vi "MeasuringDevice.Init.vi"(8 "error in (no error)":errorcluster, 11 "OPM.ThorlabsPM400":refnum<class "OPM.ThorlabsPM400.lvclass">) -> (0 "error out":errorcluster, 3 "OPM.ThorlabsPM400 out":refnum<class "OPM.ThorlabsPM400.lvclass">)   [LabVIEW 2017, in "OPM.ThorlabsPM400.lvclass"]
doc: "---------------------------------------------------------------\nJKI State Machine Objects™\nhttp://jki.net/state-machine-objects/\nCopyright (C) 2005-2015, JKI <info@jki.net>\nALL RIGHTS RESERVEDJKI State Machine Objects (SMO) 1.0.0.5\nJKI - JKI\nCopyright (c) 2016, JKI"
uses:
  OPM.ThorlabsPM400.lvclass
  D:/upwork/Laser Measurement Tool/Laser/project/Subsystems/OPM/OPM.lvclass
  Typedefs/Resource--Cluster.ctl
  OPM/OPM.lvclass
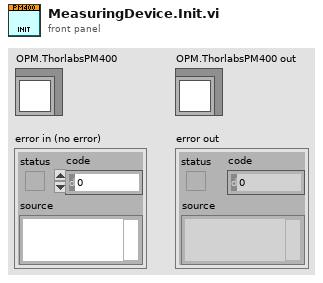
[diagram p1: front panel]
types:
  T1 = typedef "OPM.ThorlabsPM400.lvclass/Resource--Cluster.ctl" = cluster{"Instrument handle":refnum<visa-resource-name>}
  T2 = typedef "OPM.lvclass/Configuration--Cluster.ctl" = cluster{"Resource Name":string}
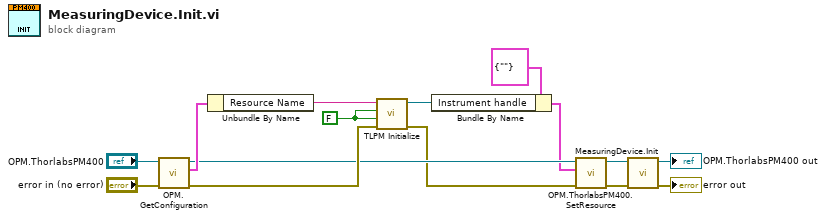
[diagram p0: block diagram]
diagram:
  w9 = FALSE ("ID Query (Do Query)")
  n1 = call "OPM.GetConfiguration.vi"("error in (no error)"="error in (no error)", "PM"="OPM.ThorlabsPM400") -> ("error out"=w8:errorcluster, "Configuration"=w11:T2, "PM out"=w5:refnum<class "OPM.ThorlabsPM400.lvclass">)  [unwired: 7 in]
  n2 = Unbundle By Name(w11) -> ("Resource Name"=w10:string)
  n3 = call <instrlib>:"TLPM Initialize.vi"("error in (no error)"=w8, "Reset Device (Reset Device)"=w9, "ID Query (Do Query)"=w9, "resource name"=w10) -> ("error out"=w3:errorcluster, "instrument handle out"=w6:refnum<visa-resource-name>)  [unwired: 6 in]
  n4 = Bundle By Name(cluster=T1 {"Instrument handle"=""} ("Resource"), "Instrument handle"=w6) -> (w4:T1)
  n5 = call "OPM.ThorlabsPM400.SetResource.vi"("error in (no error)"=w3, "Resource"=w4, "OPM.ThorlabsPM400 in"=w5) -> ("error out"=w1:errorcluster, "OPM.ThorlabsPM400 out"=w2:refnum<class "OPM.ThorlabsPM400.lvclass">)  [unwired: 7 in]
  n6 = call-parent "MeasuringDevice.Init.vi"("error in (no error)"=w1, "MeasuringDevice"=w2) -> ("error out"=→"error out":errorcluster, "MeasuringDevice out"=→"OPM.ThorlabsPM400 out":refnum<class "OPM.ThorlabsPM400.lvclass">)  [unwired: 8 in]
